vi "GetAttribute.vi"(8 "error in (no error)":errorcluster, 11 "Data_Gaze in":refnum<class "Data_Gaze.lvclass">) -> (0 "error out":errorcluster, 2 "Attribute":T1, 3 "Data_Gaze out":refnum<class "Data_Gaze.lvclass">)   [LabVIEW 2020, in "Data_Gaze.lvclass"]
uses:
  Data_Gaze.lvclass
  Attribute.vi
  Data_Gaze.lvclass/Data_Gaze.ctl
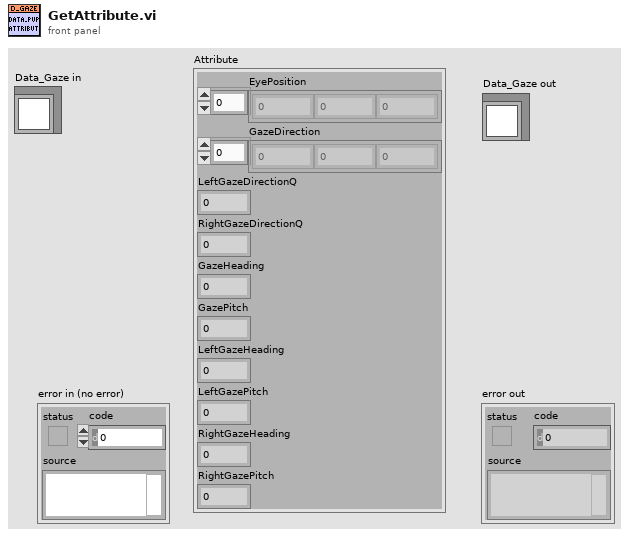
[diagram p1: front panel]
types:
  T1 = typedef "Data_Gaze.lvclass/Attribute.vi" = cluster{"EyePosition":dbl[], "GazeDirection":dbl[], "LeftGazeDirectionQ":dbl, "RightGazeDirectionQ":dbl, "GazeHeading":dbl, "GazePitch":dbl, "LeftGazeHeading":dbl, "LeftGazePitch":dbl, "RightGazeHeading":dbl, "RightGazePitch":dbl}
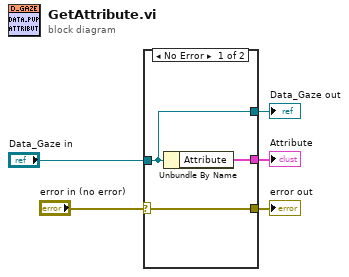
[diagram p0: block diagram]
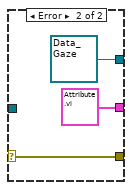
[diagram p2: hidden frame]
diagram:
  n1 = case shown="No Error" "error in (no error)" {
    selector: "error in (no error)" -> [w8 w11]
    tunnel: [w8 w11] -> w4
    tunnel: [w7 refnum<class "Data_Gaze.lvclass"> refnum ("Data_Pupil_Diameter in")] -> w3
    tunnel: "Data_Gaze in" -> [w7 _]
    tunnel: [w6 T1 {"EyePosition"=[], "GazeDirection"=[], "LeftGazeDirectionQ"=0.0, "RightGazeDirectionQ"=0.0, "GazeHeading"=0.0, "GazePitch"=0.0, "LeftGazeHeading"=0.0, "LeftGazePitch"=0.0, "RightGazeHeading"=0.0, "RightGazePitch"=0.0} ("Attribute")] -> w1
    frame No Error {
      n2 = Unbundle By Name(w7) -> ("Attribute"=w6:T1)
    }
    frame Error {
    }
  }
  "error out" <- w4
  "Data_Gaze out" <- w3
  "Attribute" <- w1
